vi "RegisterObserver.vi"(0 "reference in":refnum<class "WeatherStation.lvclass">, 2 "Observer":refnum<class "Observer.lvclass">, 5 "error in (no error)":errorcluster) -> (14 "reference out":refnum<class "WeatherStation.lvclass">, 16 "Added?":bool, 19 "error out":errorcluster)   [LabVIEW 2020, in "WeatherStation.lvclass"]
uses:
  WeatherStation.lvclass
  Observer_class/Observer.lvclass
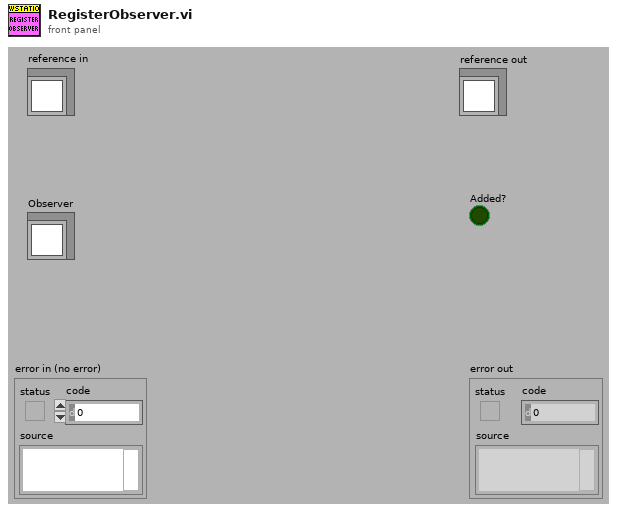
[diagram p1: front panel]
types:
  T1 = typedef "WeatherStation.lvclass/ObjectAttributes.ctl" = cluster{"WeatherData":T2, "Observers":refnum<class "Observer.lvclass">[]}
  T2 = typedef "WeatherData.ctl" = cluster{"Temperature C":dbl, "Humid %":dbl, "Pressure":dbl, "Forecast":string}
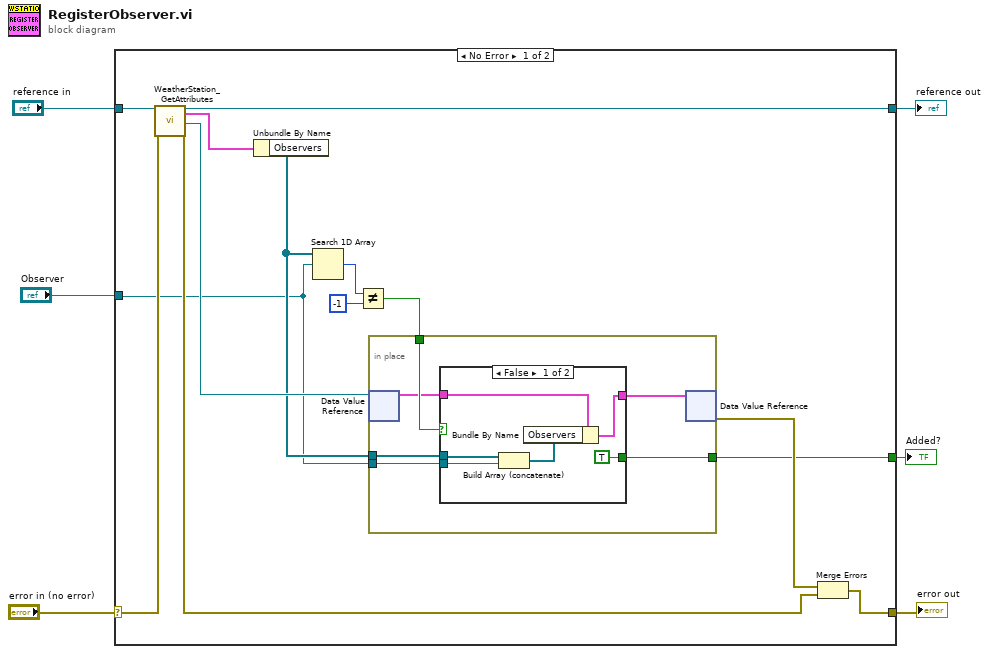
[diagram p0: block diagram]
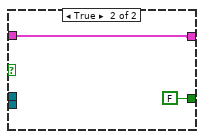
[diagram p2: hidden frame]
diagram:
  n1 = case shown="No Error" "error in (no error)" {
    selector: "error in (no error)" -> [w20 w36]
    tunnel: [w12 w36] -> w5
    tunnel: [w17 w35] -> w3
    tunnel: "reference in" -> [w18 w35]
    tunnel: "Observer" -> [w8 _]
    tunnel: [w7 _] -> w1
    frame No Error {
      n2 = call "WeatherStation_GetAttributes.vi"("reference in"=w18, "error in (no error)"=w20) -> ("reference out"=w17:refnum<class "WeatherStation.lvclass">, "Data"=w19:T1, "DataRef"=w10:refnum<data-value>, "error out"=w13:errorcluster)  [unwired: 14 in]
      n3 = Unbundle By Name(w19) -> ("Observers"=w9:refnum<class "Observer.lvclass">[])
      n4 = Search 1D Array(1D array=w9, element=w8) -> (index of element=w16:i32)  [unwired: 1 in]
      n5 = Not Equal?(x=w16, y=-1) -> (x != y?=w11:bool)
      n6 = in-place {
        in-place-border: w11 -> [w26]
        in-place-border: w9 -> [w24]
        in-place-border: w8 -> [w23]
        in-place-border: [w21] -> w7
        n7 = in-place-dvr #1(w10) -> (w25:T1)  [unwired: 1 out]
        n8 = case shown="False" w26 {
          tunnel: w25 -> [w32 w34]
          tunnel: w24 -> [w31 _]
          tunnel: w23 -> [w30 _]
          tunnel: [w28 w34] -> w22
          tunnel: [TRUE FALSE] -> w21
          frame False {
            n9 = Build Array (concatenate)(w31, w30) -> (w29:refnum<class "Observer.lvclass">[])
            n10 = Bundle By Name(cluster=w32, "Observers"=w29) -> (w28:T1)
          }
          frame True {
          }
        }
        n11 = in-place-dvr #1(w22) -> (w14:errorcluster)  [unwired: 1 out]
      }
      n12 = Merge Errors(w14, w13) -> (w12:errorcluster)
    }
    frame Error {
    }
  }
  "error out" <- w5
  "reference out" <- w3
  "Added?" <- w1
